vi "PicoScope5000aOpen.vi"(0 "USB 3.0 device on non-USB 3.0 Port control":bool, 7 "Serial Number":string, 8 "USB Powered control":bool, 9 "Resolution":i32(ring) items=["8-bit", "12-bit", "14-bit", "15-bit (max. 2 ch.)", "16-bit (max. 1 ch.)"], 10 "Use Serial Number":bool, 11 "error in (no error)":errorcluster) -> (1 "USB Powered":bool, 2 "handle":i16, 3 "error out":errorcluster, 4 "Max ADC value":i16, 5 "USB 3.0 device on non-USB 3.0 Port":bool, 6 "Device Info":T1)   [LabVIEW 2009]
doc: "This VI opens a PicoScope 3000a/b and returns a handle to the device."
uses:
  ps5000a.dll
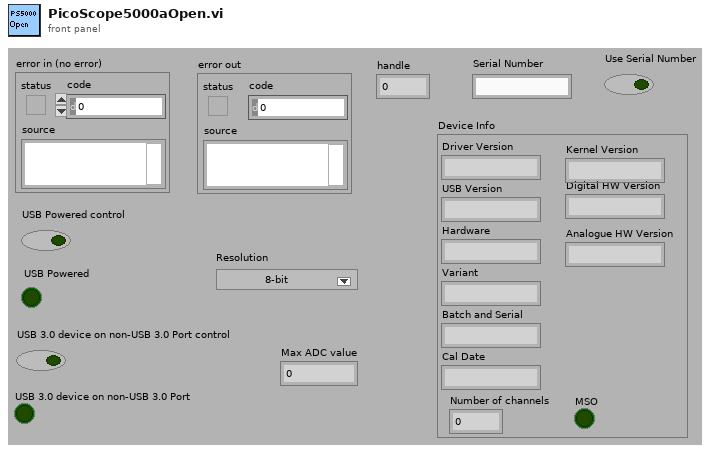
[diagram p1: front panel]
types:
  T1 = cluster{"Driver Version":string, "USB Version":string, "Hardware":string, "Variant":string, "Batch and Serial":string, "Cal Date":string, "Kernel Version":string, "Digital HW Version":string, "Analogue HW Version":string, "MSO":bool, "Number of channels":i16}
  T2 = cluster{"Driver Version":string, "USB Version":string, "Hardware":string, "Variant":string, "Batch and Serial":string, "Cal Date":string, "Kernel Version":string, "Digital HW Version":string, "Analogue HW Version":string, "Firmware 1":string, "Firmware 2":string}
  T3 = cluster{"Driver Version":string, "USB Version":string, "Hardware":string, "Variant":string, "Batch and Serial":string, "Cal Date":string, "Kernel Version":string, "Digital HW Version":string, "Analogue HW Version":string, bool, i16}
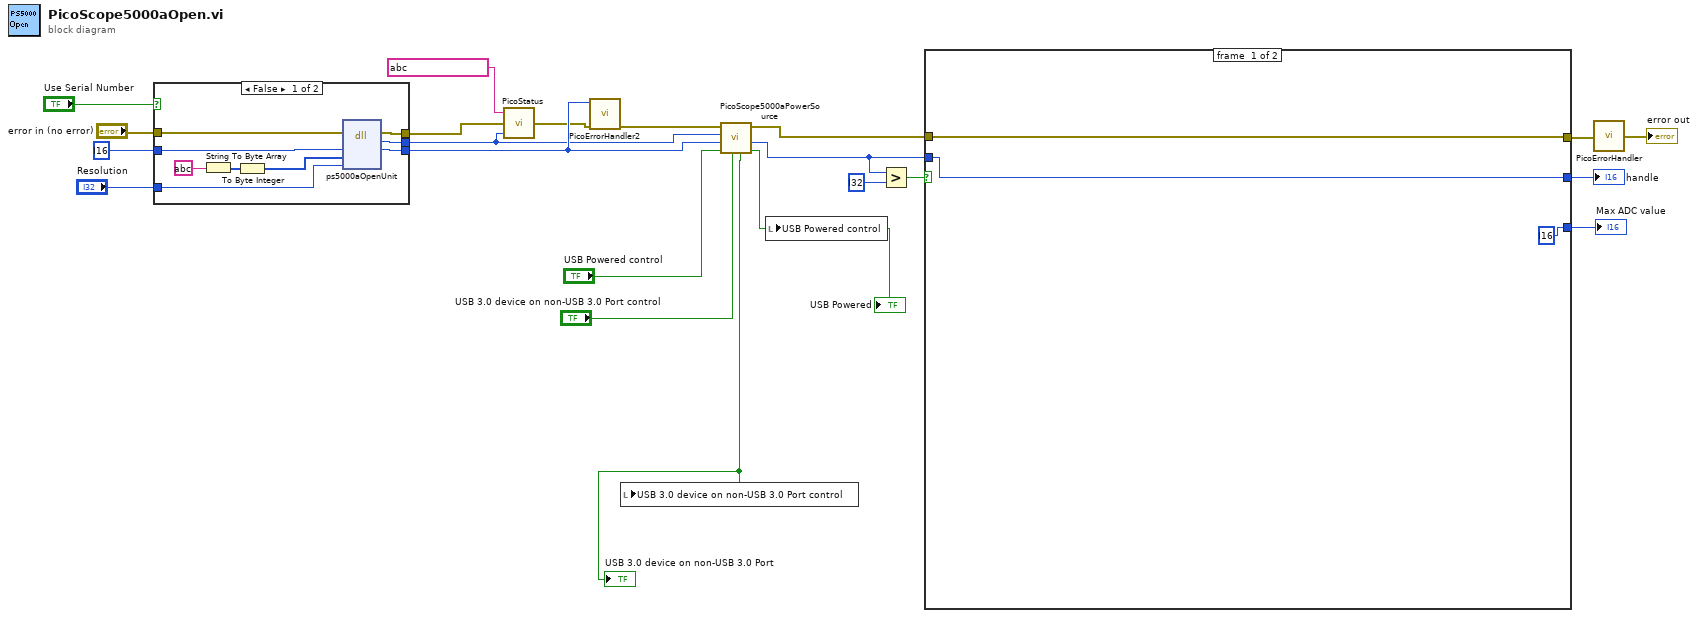
[diagram p0: block diagram]
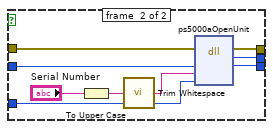
[diagram p2: hidden frame]
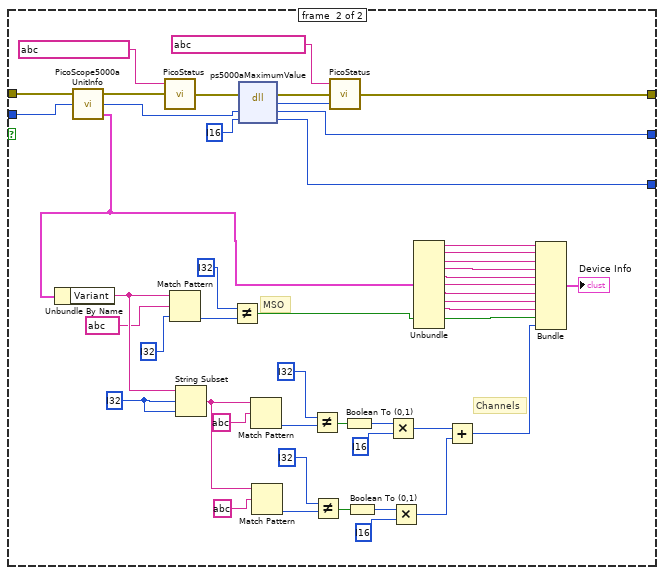
[diagram p3: hidden frame]
diagram:
  n1 = case shown="False" "Use Serial Number" {
    tunnel: "error in (no error)" -> [w31 w36]
    tunnel: i16 ? ("handle") -> [w26 w37]
    tunnel: [w30 w40] -> w4
    tunnel: [w29 w39] -> w2
    tunnel: [w28 w38] -> w6
    tunnel: "Resolution" -> [w27 w35]
    frame #0 {
      n2 = String To Byte Array(string=string ?) -> (unsigned byte array=w24:u8[])
      n3 = To Byte Integer(number=w24) -> (8bit integer=w23:i8[])
      n4 = dll-call lib="ps5000a.dll" fn="ps5000aOpenUnit" ("ps3000.dll:_ps3000_open_unit@0")(error in=w31, "handle"=w26, "serial"=w23, "resolution"=w27) -> (error out=w30:errorcluster, "PICO_STATUS"=w29:u32, "handle"=w28:i16)  [unwired: 4 in, 1 out]
    }
    frame #1 {
      n5 = To Upper Case(1:"Serial Number") -> (0:w33:string)
      n6 = call <vilib>:"Trim Whitespace.vi"("string"=w33) -> ("trimmed string"=w32:string)  [unwired: 1 in]
      n7 = dll-call lib="ps5000a.dll" fn="ps5000aOpenUnit" ("ps3000.dll:_ps3000_open_unit@0")(error in=w36, "handle"=w37, "serial"=w32, "resolution"=w35) -> (error out=w40:errorcluster, "PICO_STATUS"=w39:u32, "handle"=w38:i16)  [unwired: 4 in, 1 out]
    }
  }
  n8 = call "PicoStatus.vi"("PICO STATUS"=w2, "error in"=w4, "source"=string ?) -> ("error out"=w5:errorcluster)
  n9 = call "PicoErrorHandler2.vi"("error in (no error)"=w5, "handle In"=w6) -> ("error out"=w7:errorcluster)  [unwired: 9 in]
  n10 = call "PicoScope5000aPowerSource.vi"("USB 3.0 on non-USB 3.0 port control"="USB 3.0 device on non-USB 3.0 Port control", "USB Powered control"="USB Powered control", "handle in"=w6, "PICO STATUS IN"=w2, "error in (no error)"=w7) -> ("USB Powered"=w18:bool, "handle out"=w14:i16, "error out"=w1:errorcluster, "USB 3.0 on non-USB 3.0 Port"=w8:bool)  [unwired: 2 in, 1 out]
  "USB Powered" <- w18
  "USB 3.0 device on non-USB 3.0 Port" <- w8
  n11 = local write "USB 3.0 device on non-USB 3.0 Port control"(w8) -> ()
  n12 = local write "USB Powered control"(w18) -> ()
  n13 = Greater?(x=w14, y=i32 ?) -> (0:w15:bool)
  n14 = case shown="True" w15 {
    tunnel: w14 -> [w42 w90]
    tunnel: w1 -> [w43 w89]
    tunnel: [w43 w49] -> w17
    tunnel: [w42 w47] -> w16
    tunnel: [i16 ? ("value") w45] -> w10
    frame #0 {
    }
    frame #1 {
      w77 = i32 ? ("offset (0)")
      # "MSO"
      # "Channels"
      n15 = call "PicoScope5000aUnitInfo.vi"("handle in"=w90, "error in (no error)"=w89) -> ("Unit Info"=w53:T2, "handle out"=w51:i16, "error out"=w88:errorcluster)  [unwired: 1 in]
      n16 = Unbundle By Name(w53) -> ("Variant"=w73:string)
      n17 = call "PicoStatus.vi"("error in"=w88, "source"=string ?) -> ("error out"=w52:errorcluster)  [unwired: 1 in]
      n18 = Match Pattern(string=w73, regular expression=string ?, offset (0)=i32 ?) -> (offset past match=w70:i32)  [unwired: 3 out]
      n19 = String Subset(string=w73, offset (0)=w77, length (rest)=w77) -> (substring=w64:string)
      n20 = Not Equal?(x=i32 ?, y=w70) -> (x != y?=w68:bool)
      n21 = dll-call lib="ps5000a.dll" fn="ps5000aMaximumValue"(error in=w52, "handle"=w51, "value"=i16 ?) -> (error out=w50:errorcluster, "PICO_STATUS"=w48:u32, "handle"=w47:i16, "value"=w45:i16)  [unwired: 2 in, 1 out]
      n22 = Match Pattern(string=w64, regular expression=string ?) -> (offset past match=w75:i32)  [unwired: 1 in, 3 out]
      n23 = Match Pattern(string=w64, regular expression=string ?) -> (offset past match=w66:i32)  [unwired: 1 in, 3 out]
      n24 = Not Equal?(x=i32 ?, y=w75) -> (x != y?=w60:bool)
      n25 = Not Equal?(x=i32 ?, y=w66) -> (x != y?=w56:bool)
      n26 = call "PicoStatus.vi"("PICO STATUS"=w48, "error in"=w50, "source"=string ?) -> ("error out"=w49:errorcluster)
      n27 = Boolean To (0,1)(Boolean=w60) -> (0, 1=w59:i16)
      n28 = Boolean To (0,1)(Boolean=w56) -> (0, 1=w57:i16)
      n29 = Multiply(x=w59, y=i16 ?) -> (x*y=w63:i16)
      n30 = Multiply(x=w57, y=i16 ?) -> (x*y=w55:i16)
      n31 = Unbundle(w53) -> ("Driver Version"=w86:string, "USB Version"=w85:string, "Hardware"=w84:string, "Variant"=w83:string, "Batch and Serial"=w82:string, "Cal Date"=w81:string, "Kernel Version"=w80:string, "Digital HW Version"=w79:string, "Analogue HW Version"=w78:string)  [unwired: 2 out]
      n32 = Add(x=w63, y=w55) -> (x+y=w62:i16)
      n33 = Bundle("Driver Version"=w86, "USB Version"=w85, "Hardware"=w84, "Variant"=w83, "Batch and Serial"=w82, "Cal Date"=w81, "Kernel Version"=w80, "Digital HW Version"=w79, "Analogue HW Version"=w78, w68, w62) -> (→"Device Info":T3)  [unwired: 1 in]
    }
  }
  "handle" <- w16
  "Max ADC value" <- w10
  n34 = call "PicoErrorHandler.vi"("error in"=w17) -> ("error out"=→"error out":errorcluster)
